vi "GT_GetAxisEncPos.vi"(6 "Axis in":T1=1 items=["Axis Control"=0, "Axis 1"=1, "Axis 2"=2, "Axis 3"=3, "Axis 4"=4, "Axis 5"=5, "Axis 6"=6, "Axis 7"=7, "Axis 8"=8, "Vector Space Control"=16, "Vector Space 1"=17, "Vector Space 2"=18, "Vector Space 3"=19, "Vector Space 4"=20], 7 "rtn_In":cluster{"rtn":i16, "Func":string}) -> (0 "pClock":u32, 1 "pValue":dbl, 2 "axis out":i16, 3 "rtn_Out":cluster{"rtn":i16, "Func":string})   [LabVIEW 2014]
uses:
  <vilib>/Motion/FlexMotion/CustomControls/CustomControls.llb/AxisOrVectorSpaceControl To Control.flx
  VC6/gts.dll
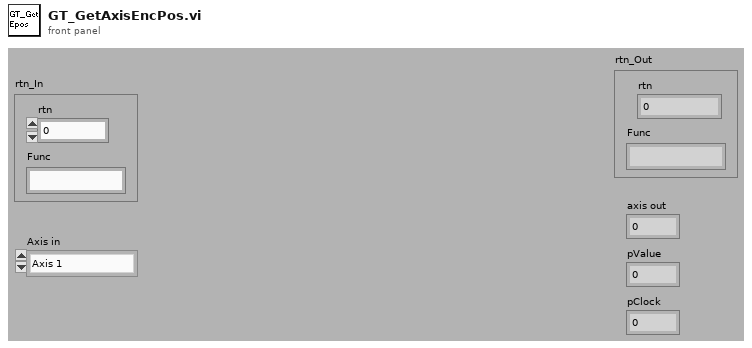
[diagram p1: front panel]
types:
  T1 = typedef "AxisOrVectorSpaceControl To Control.flx" = u16
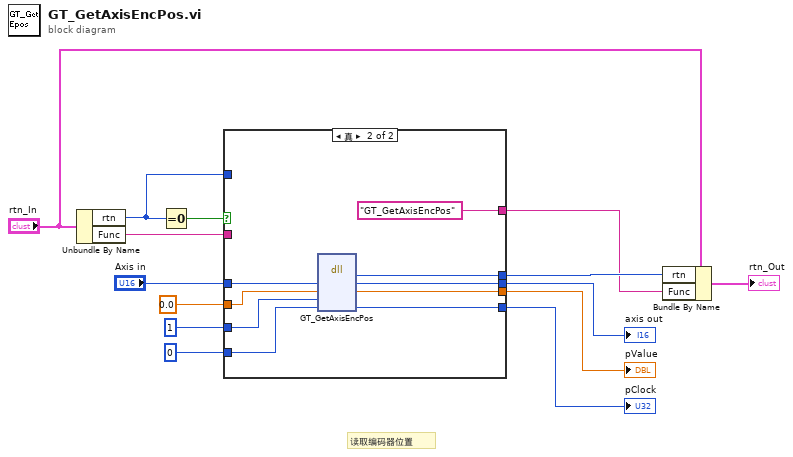
[diagram p0: block diagram]
diagram:
  # "读取编码器位置"
  n1 = Unbundle By Name("rtn_In") -> ("rtn"=w2:i16, "Func"=w1:string)
  n2 = Equal To 0?(x=w2) -> (x = 0?=w14:bool)
  n3 = case shown="真" w14 {
    tunnel: [w16 w28] -> w11
    tunnel: [w15 "GT_GetAxisEncPos" ("Func")] -> w10
    tunnel: 0.0 ("pValue") -> [w19 w26]
    tunnel: i16 1 ("count") -> [_ w25]
    tunnel: u32 0 ("pClock") -> [w18 w24]
    tunnel: [w17 w23] -> w6
    tunnel: [w19 w22] -> w5
    tunnel: [w18 w21] -> w4
    tunnel: "Axis in" -> [w17 w20]
    tunnel: w2 -> [w16 _]
    tunnel: w1 -> [w15 _]
    frame False {
    }
    frame True {
      n4 = dll-call lib="PTH2Fabs DNewGTS AC-800LWin7版源程序-20170926gts85VC6gts.dll" fn="GT_GetAxisEncPos"("axis"=w20, "pValue"=w26, "count"=w25, "pClock"=w24) -> ("rtn"=w28:i16, "axis"=w23:i16, "pValue"=w22:dbl, "pClock"=w21:u32)  [unwired: 4 in, 2 out]
    }
  }
  "axis out" <- w6
  "pValue" <- w5
  "pClock" <- w4
  n5 = Bundle By Name(cluster="rtn_In", "rtn"=w11, "Func"=w10) -> (→"rtn_Out":cluster{"rtn":i16, "Func":string})
